vi "getFingerprint.vi"(0 "MoAgSy_GPG in":refnum<class "MoAgSy_GPG.lvclass">, 1 "options file":path, 2 "keyringfile":path, 3 "Sec keyringfile":path, 5 "error in (no error)":errorcluster, 6 "key-id":string, 8 "Trust DB":path) -> (10 "dup Trust DB":path, 12 "fingerprint":string, 14 "dup MoAgSy_GPG":refnum<class "MoAgSy_GPG.lvclass">, 15 "dup options file":path, 16 "dup keyringfile":path, 17 "dup Sec keyringfile":path, 19 "error out":errorcluster)   [LabVIEW 2009, in "MoAgSy.lvlib" / "MoAgSy_GPG.lvclass"]
doc: "Get fingerprint of Key-ID. If no Key-ID is set, the Objects Fingerprint will be returned."
uses:
  MoAgSy_GPG.lvclass
  HGF_GPG/HGF_GPG.lvclass/HGF_GPG.lvclass
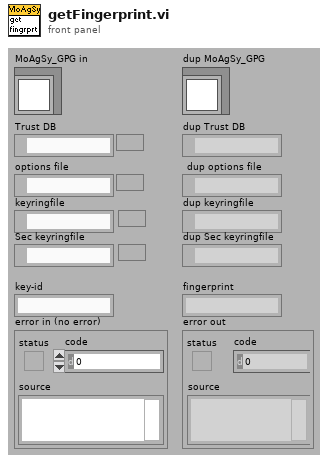
[diagram p1: front panel]
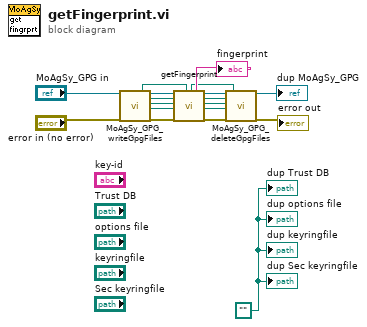
[diagram p0: block diagram]
diagram:
  w17 = path ""
  n1 = call "MoAgSy_GPG_writeGpgFiles.vi"("MoAgSy_GPG"="MoAgSy_GPG in", "error in (no error)"="error in (no error)") -> ("trust db file"=w1:path, "dup MoAgSy_GPG"=w15:refnum<class "MoAgSy_GPG.lvclass">, "options file"=w2:path, "keyring file"=w3:path, "sec keyring file"=w4:path, "error out"=w13:errorcluster)  [unwired: 12 out]
  n2 = call-parent "getFingerprint.vi"("HGF_GPG in"=w15, "options file"=w2, "keyringfile"=w3, "Sec keyringfile"=w4, "error in (no error)"=w13, "Trust DB"=w1) -> ("dup Trust DB"=w8:path, "fingerprint"=→"fingerprint":string, "dup HGF_GPG"=w10:refnum<class "MoAgSy_GPG.lvclass">, "dup options file"=w7:path, "dup keyringfile"=w6:path, "dup Sec keyringfile"=w5:path, "error out"=w12:errorcluster)  [unwired: 1 in, 6 out]
  n3 = call "MoAgSy_GPG_deleteGpgFiles.vi"("MoAgSy_GPG"=w10, "options file"=w7, "keyringfile"=w6, "Sec keyringfile"=w5, "error in (no error)"=w12, "Trust DB"=w8) -> ("dup MoAgSy_GPG"=→"dup MoAgSy_GPG":refnum<class "MoAgSy_GPG.lvclass">, "error out"=→"error out":errorcluster)  [unwired: 12 out]
  "dup keyringfile" <- w17
  "dup options file" <- w17
  "dup Sec keyringfile" <- w17
  "dup Trust DB" <- w17
